vi "Find_Number_LineMARVIN.vi"(4 "Test Paragraph":string, 5 "error in":errorcluster, 7 "TableIn":refnum<vi>, 8 "Row Headers[]":string[](array[string])) -> (0 "error out":errorcluster, 1 "1 line Test ?":bool, 2 "Found":bool, 3 "Line number":i32)   [LabVIEW 2017]
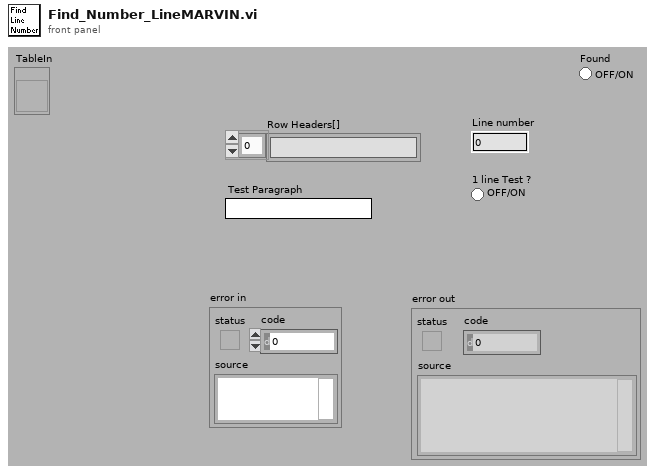
[diagram p1: front panel]
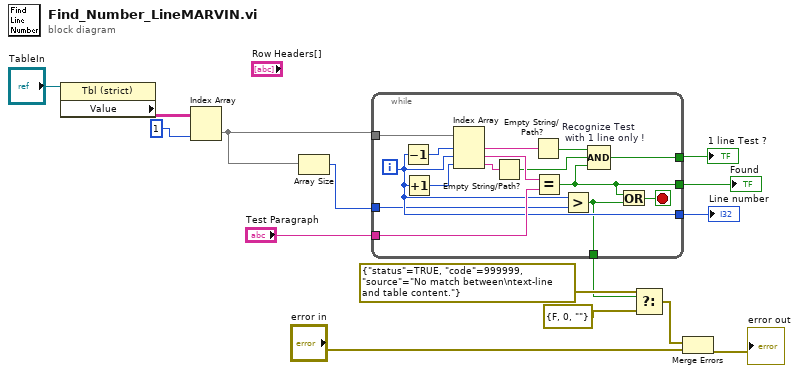
[diagram p0: block diagram]
diagram:
  n1 = property class="Tbl (strict)"(reference="TableIn") -> ("Value"=w4:string[][])  [unwired: 1 in, 2 out]
  n2 = Index Array(array=w4, index (col)=1 ("disabled index (col)")) -> (element=w2:string[])  [unwired: 1 in]
  n3 = Array Size(array=w2) -> (size(s)=w12:i32)
  n4 = while {
    tunnel: "Test Paragraph" -> [w30]
    tunnel: w2 -> [w29]
    tunnel: [w20] -> w14
    tunnel: [w19] -> w15
    tunnel: w12 -> [w18]
    tunnel: [w17] -> w8
    tunnel: [w16] -> w5
    i -> [w19]
    stop <- w21 stop-if-true
    n5 = Decrement(x=w19) -> (x-1=w28:i32)
    n6 = Increment(x=w19) -> (x+1=w27:i32)
    n7 = Index Array(array=w29, index #1=w28, index #2=w19, index #3=w27) -> (element #1=w25:string, element #2=w26:string, element #3=w24:string)
    n8 = Empty String/Path?(string/path=w24) -> (empty?=w22:bool)
    n9 = Empty String/Path?(string/path=w25) -> (empty?=w23:bool)
    n10 = Equal?(x=w26, y=w30) -> (x = y?=w16:bool)
    n11 = Greater?(x=w19, y=w18) -> (0:w17:bool)
    n12 = Compound Arithmetic op=AND "Recognize Test \n with 1 line only !"(w23, w22, w16) -> (w20:bool)
    n13 = Or(x=w16, y=w17) -> (x .or. y?=w21:bool)
  }
  "Line number" <- w15
  "1 line Test ?" <- w14
  "Found" <- w5
  n14 = Select(t=errorcluster {"status"=TRUE, "code"=999999, "source"="No match between\ntext-line and table content."} ("error in 1 (no error)"), s=w8, f=errorcluster {"status"=FALSE, "code"=0, "source"=""}) -> (s? t:f=w6:errorcluster)
  n15 = Merge Errors(w6, "error in") -> (→"error out":errorcluster)
